vi "Cluster to Graph.vi"() -> ()   [LabVIEW 2022 SP3]
panel:
  out "Waveform Graph":cluster{"x0":dbl, "Delta x":dbl, "Array":dbl[]}(graph)
  in  "Cluster":T1
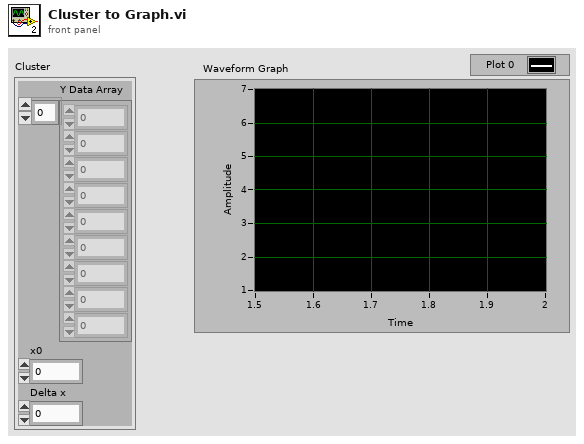
[diagram p1: front panel]
types:
  T1 = cluster{"Y Data Array":dbl[], "x0":dbl, "Delta x":dbl}
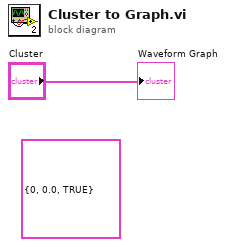
[diagram p0: block diagram]
diagram:
  (unwired) cluster{i32, dbl, bool} {0, 0.0, TRUE}
  "Waveform Graph" <- "Cluster"
